vi "Hitrap_DiagnosticBox.GoToPosition.vi"(0 "i ref in":refnum<vi>, 2 "Timeout":i32, 3 "Axis":i32, 4 "StepsFromPosition":dbl, 5 "error in":errorcluster) -> (14 "i ref out":refnum<vi>, 19 "error out":errorcluster)   [LabVIEW 2014, in "Hitrap_DiagnosticBox.lvlib"]
doc: "perform a reference move"
uses:
  Hitrap_DiagnosticBox.lvlib
  CSCore/CSApplicationBaseClasses/MotorBase/MotorBase.directionType.ctl
  CSCore/CSApplicationBaseClasses/MotorBase/MotorBase.serviceType.ctl
  CSMotion/NanotecSMCPD/NanotecSMCPD.lvlib
  CSCore/CSApplicationBaseClasses/MotorBase/MotorBase.lvlib
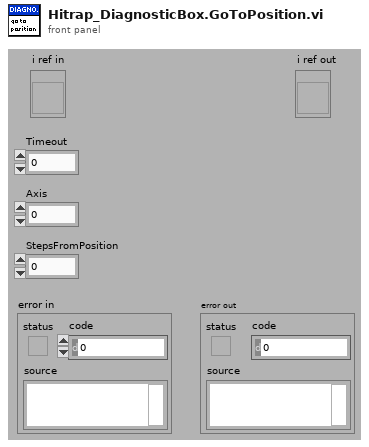
[diagram p1: front panel]
types:
  T1 = typedef "MotorBase.lvlib/MotorBase.serviceType.ctl" = enum16{"onOff", "startVelocity", "stopVelocity", "acceleration", "rangeMin", "rangeMax", "status", "position"}
  T2 = typedef "MotorBase.lvlib/MotorBase.directionType.ctl" = enum16{"unknown", "update actual value", "update nominal value", "update both"}
  T3 = typedef "NanotecSMCPD.lvlib/NanotecSMCPD.i attribute.ctl" = cluster{"referencing":bool[], "stop":bool[], "AutoHalt ID":i32, "MethodQueue":refnum<queue>, "Referenced1Time?":bool[], "LastCommand ID":i32}
  T4 = typedef "MotorBase.lvlib/MotorBase.i attribute.ctl" = cluster{"defaultAxisIndex":i32, "logicalName":string[], "nOfAxes":i32, "physicalName":string[], "scaling":dbl[], "units":string[], "defaulAxisIndexID":i32, "logicalNameID":i32, "nOfAxesID":i32, "physicalNameID":i32, "unitID":i32, "actValues":T5, "nomValues":T5}
  T5 = typedef "MotorBase.lvlib/MotorBase.parameters.ctl" = cluster{"services":cluster{"onOff":bool[], "startVelocity":dbl[], "stopVelocity":dbl[], "acceleration":dbl[], "rangeMin":dbl[], "rangeMax":dbl[], "status":T6[], "position":dbl[]}, "serviceIDs":cluster{"onOffID":i32, "startVelocityID":i32, "stopVelocityID":i32, "accelerationID":i32, "rangeMinID":i32, "rangeMaxID":i32, "statusID":i32, "positionID":i32}}
  T6 = typedef "MotorBase.lvlib/MotorBase.statusType.ctl" = u32
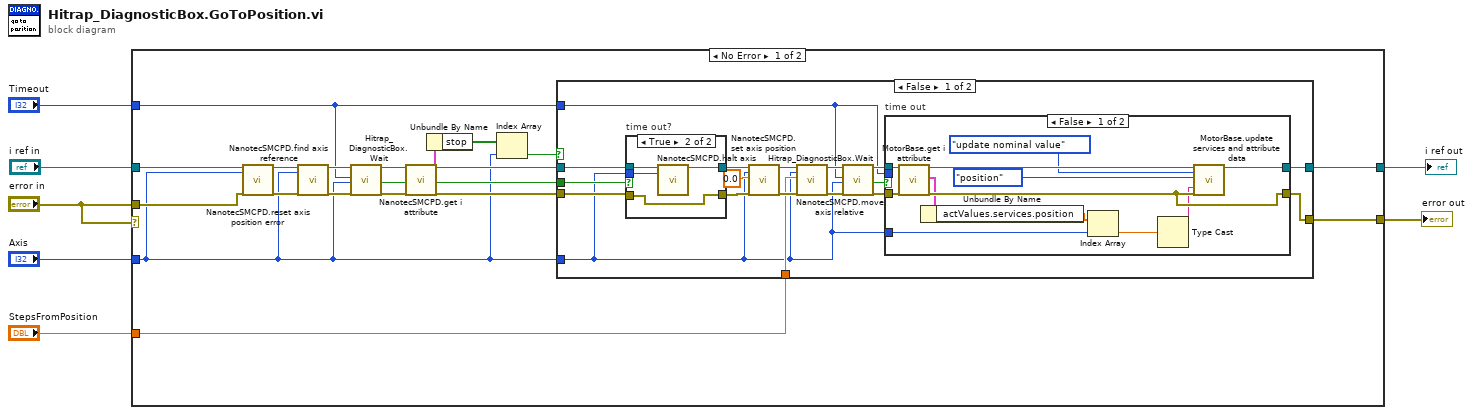
[diagram p0: block diagram]
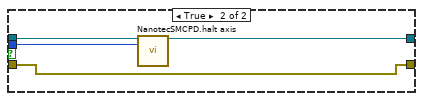
[diagram p2: hidden frame]
diagram:
  n1 = case shown="No Error" "error in" {
    tunnel: "i ref in" -> [w26 w69]
    tunnel: [w24 w69] -> w6
    tunnel: "error in" -> [w23 w70]
    tunnel: [w21 w70] -> w5
    tunnel: "Axis" -> [w8 _]
    tunnel: "Timeout" -> [w16 _]
    tunnel: "StepsFromPosition" -> [w20 _]
    frame No Error {
      n2 = call "NanotecSMCPD.reset axis position error.vi"("i ref in"=w26, "axis"=w8, "error in (no error)"=w23) -> ("i ref out"=w25:refnum<vi>, "error out"=w22:errorcluster)  [unwired: 15 in]
      n3 = call "NanotecSMCPD.find axis reference.vi"("i ref in"=w25, "axis"=w8, "error in (no error)"=w22) -> ("i ref out"=w17:refnum<vi>, "error out"=w18:errorcluster)  [unwired: 14 in, 1 out]
      n4 = call "Hitrap_DiagnosticBox.Wait.vi"("i ref in"=w17, "Timeout"=w16, "Axis"=w8, "error in"=w18) -> ("i ref out"=w15:refnum<vi>, "Timeout?"=w19:bool, "error out"=w13:errorcluster)  [unwired: 13 in]
      n5 = call "NanotecSMCPD.get i attribute.vi"("i ref in"=w15, "error in (no error)"=w13) -> ("i ref out"=w14:refnum<vi>, "i attribute"=w11:T3, "error out"=w12:errorcluster)  [unwired: 15 in]
      n6 = Unbundle By Name(w11) -> ("stop"=w10:bool[])
      n7 = Index Array(array=w10, index=w8) -> (element=w9:bool)
      n8 = case shown="False" w9 {
        tunnel: [w42 w68] -> w24
        tunnel: [w39 w67] -> w21
        tunnel: w20 -> [w37 _]
        tunnel: w14 -> [w36 w68]
        tunnel: w19 -> [w35 _]
        tunnel: w12 -> [w34 w67]
        tunnel: w8 -> [w27 _]
        tunnel: w16 -> [w28 _]
        frame False {
          n9 = case "time out?" shown="True" w35 {
            tunnel: w36 -> [w62 w66]
            tunnel: [w62 w65] -> w44
            tunnel: [w61 w63] -> w41
            tunnel: w27 -> [_ w64]
            tunnel: w34 -> [w61 w63]
            frame False {
            }
            frame True {
              n10 = call "NanotecSMCPD.halt axis.vi"("i ref in"=w66, "axis"=w64) -> ("i ref out"=w65:refnum<vi>)  [unwired: 15 in, 2 out]
            }
          }
          n11 = call "NanotecSMCPD.set axis position.vi"("i ref in"=w44, "axis"=w27, "position"=0.0, "error in (no error)"=w41) -> ("i ref out"=w43:refnum<vi>, "error out"=w40:errorcluster)  [unwired: 13 in, 1 out]
          n12 = call "NanotecSMCPD.move axis relative.vi"("i ref in"=w43, "axis"=w27, "relPosition"=w37, "error in (no error)"=w40) -> ("i ref out"=w33:refnum<vi>, "error out"=w32:errorcluster)  [unwired: 13 in, 1 out]
          n13 = call "Hitrap_DiagnosticBox.Wait.vi"("i ref in"=w33, "Timeout"=w28, "Axis"=w27, "error in"=w32) -> ("i ref out"=w31:refnum<vi>, "Timeout?"=w29:bool, "error out"=w30:errorcluster)  [unwired: 13 in]
          n14 = case "time out" shown="False" w29 {
            tunnel: w31 -> [w56 w60]
            tunnel: [w53 w59] -> w42
            tunnel: w30 -> [w55 w57]
            tunnel: [w52 w57] -> w39
            tunnel: w28 -> [_ w58]
            tunnel: w27 -> [w45 _]
            frame False {
              n15 = call "MotorBase.get i attribute.vi"("i ref in"=w56, "error in (no error)"=w55) -> ("i ref out"=w54:refnum<vi>, "i attribute"=w49:T4, "error out"=w52:errorcluster)  [unwired: 15 in]
              n16 = Unbundle By Name(w49) -> ("actValues.services.position"=w47:dbl[])
              n17 = Index Array(array=w47, index=w45) -> (element=w46:dbl)
              n18 = Type Cast(x=w46) -> (*(type *) &x=w48:string)  [unwired: 1 in]
              n19 = call "MotorBase.update services and attribute data.vi"("i ref in"=w54, "direction"=MotorBase.directionType."update nominal value", "service"=MotorBase.serviceType."position", "value"=w48, "error in (no error)"=w52) -> ("i ref out"=w53:refnum<vi>)  [unwired: 12 in, 2 out]
            }
            frame True {
              n20 = call "NanotecSMCPD.halt axis.vi"("i ref in"=w60, "axis"=w58) -> ("i ref out"=w59:refnum<vi>)  [unwired: 15 in, 2 out]
            }
          }
        }
        frame True {
        }
      }
    }
    frame Error {
    }
  }
  "error out" <- w5
  "i ref out" <- w6
